vi "Water box.vi"() -> ()   [LabVIEW 2018]
panel:
  out "Pump":bool
  out "Level 2":bool
  out "Level 1":bool
  in  "stop":bool
  out "Tank":dbl(slide) scale=0.0..100.0
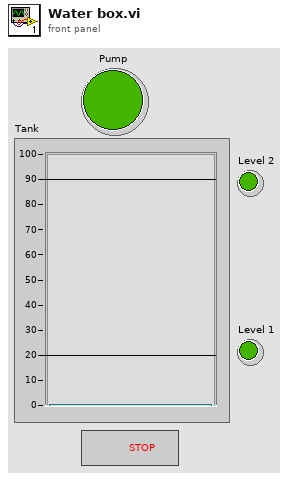
[diagram p1: front panel]
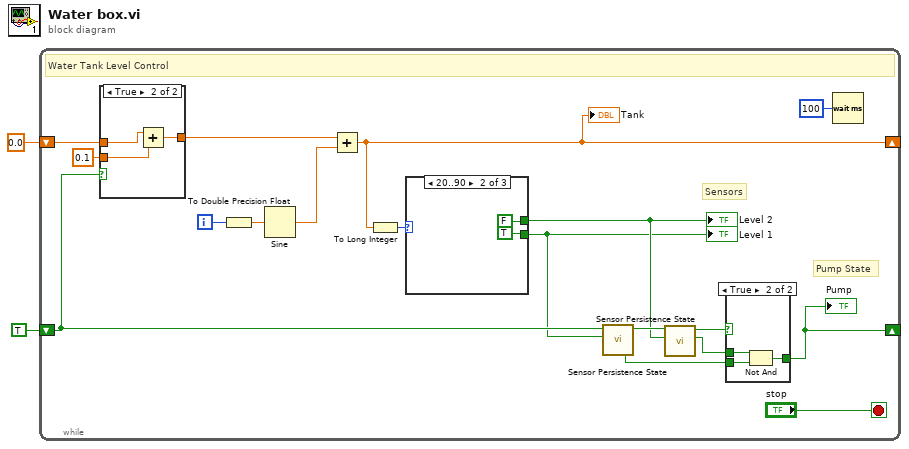
[diagram p0: block diagram]
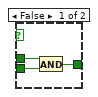
[diagram p2: hidden frame]
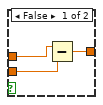
[diagram p3: hidden frame]
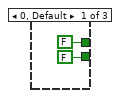
[diagram p4: hidden frame]
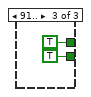
[diagram p5: hidden frame]
diagram:
  n1 = while {
    shift-right: [w14] -> _
    shift-left: TRUE -> [w13]
    shift-right: [w6] -> _
    shift-left: 0.0 -> [w15]
    i -> [w18]
    stop <- "stop" stop-if-true
    # "Pump State"
    # "Sensors"
    # "Water Tank Level Control"
    n2 = case shown="True" w13 {
      tunnel: [w29 w32] -> w4
      tunnel: w15 -> [w28 w31]
      tunnel: 0.1 ("x") -> [w27 w30]
      frame False {
        n3 = Subtract(x=w28, y=w27) -> (x-y=w29:dbl)
      }
      frame True {
        n4 = Add(x=w31, y=w30) -> (x+y=w32:dbl)
      }
    }
    n5 = To Double Precision Float(number=w18) -> (double precision float=w16:dbl)
    n6 = Sine(x=w16) -> (sin(x)=w5:dbl)
    n7 = Add(x=w4, y=w5) -> (x+y=w6:dbl)
    "Tank" <- w6
    n8 = To Long Integer(number=w6) -> (32bit integer=w17:i32)
    n9 = case shown="20..90" w17 {
      tunnel: [FALSE TRUE TRUE] -> w9
      tunnel: [FALSE FALSE TRUE] -> w10
      frame 0, Default {
      }
      frame 20..90 {
      }
      frame 91.. {
      }
    }
    "Level 1" <- w9
    "Level 2" <- w10
    n10 = call "Sensor Persistence State.vi"("Sensor"=w9, "Pump State in"=w13) -> ("Persistent State"=w7:bool, "Pump State out"=w12:bool)  [unwired: 8 in]
    n11 = call "Sensor Persistence State.vi"("Sensor"=w10, "Pump State in"=w12) -> ("Persistent State"=w8:bool, "Pump State out"=w11:bool)  [unwired: 8 in]
    n12 = case shown="True" w11 {
      tunnel: w8 -> [w22 w26]
      tunnel: [w23 w25] -> w14
      tunnel: w7 -> [w21 w24]
      frame False {
        n13 = And(x=w22, y=w21) -> (x .and. y?=w23:bool)
      }
      frame True {
        n14 = Not And(1:w24, 2:w26) -> (0:w25:bool)
      }
    }
    "Pump" <- w14
    n15 = Wait (ms)(milliseconds to wait=u32 100) -> ()  [unwired: 1 out]
  }
